vi "Get method name.vi"(8 "error in (no error)":errorcluster, 11 "VI in":refnum<vi>) -> (0 "error out":errorcluster, 1 "Body":T1, 3 "VI out":refnum<vi>)   [LabVIEW 2018]
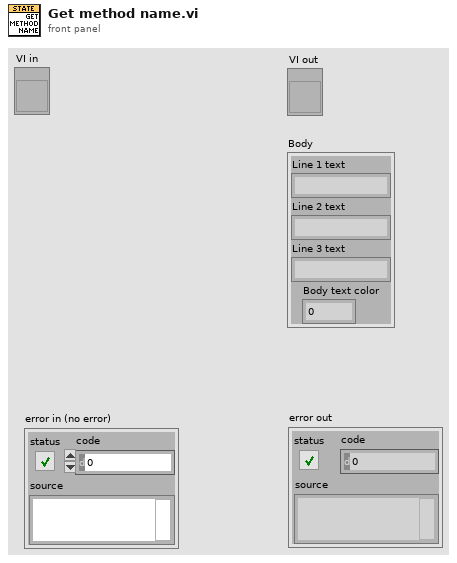
[diagram p1: front panel]
types:
  T1 = cluster{"Line 1 text":string, "Line 2 text":string, "Line 3 text":string, "Body text color":u32}
  T2 = cluster{"[0]":string, "[1]":string, "[2]":string}
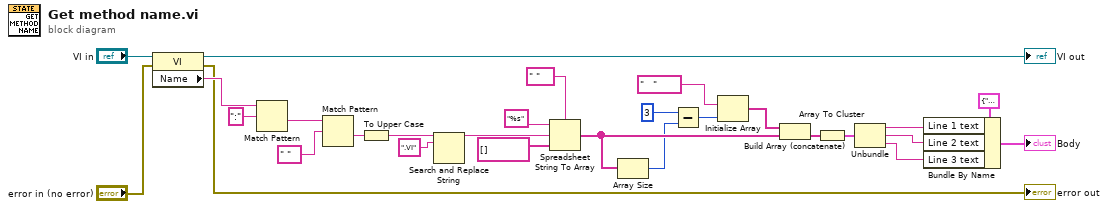
[diagram p0: block diagram]
diagram:
  n1 = property class="VI"(reference="VI in", error in="error in (no error)") -> (reference out=→"VI out":refnum<vi>, error out=→"error out":errorcluster, "Name"=w17:string)
  n2 = Match Pattern(string=w17, regular expression=":") -> (after substring=w19:string)  [unwired: 1 in, 3 out]
  n3 = Match Pattern(string=w19, regular expression=" ") -> (after substring=w20:string)  [unwired: 1 in, 3 out]
  n4 = To Upper Case(1:w20) -> (0:w22:string)
  n5 = Search and Replace String(input string=w22, search string=".VI") -> (result string=w27:string)  [unwired: 6 in, 3 out]
  n6 = Spreadsheet String To Array(delimiter (Tab)=" " ("search string"), format string="%s", spreadsheet string=w27, array type (2D Dbl)=string[] []) -> (array=w11:string[])
  n7 = Array Size(array=w11) -> (size(s)=w5:i32)
  n8 = Subtract(x=3, y=w5) -> (x-y=w4:i32)
  n9 = Initialize Array("   " ("search string"), w4) -> (w1:string[])
  n10 = Build Array (concatenate)(w1, w11) -> (w2:string[])
  n11 = Array To Cluster(array=w2) -> (cluster=w10:T2)
  n12 = Unbundle(w10) -> ("[0]"=w9:string, "[1]"=w8:string, "[2]"=w7:string)
  n13 = Bundle By Name(cluster=T1 {"Line 1 text"="", "Line 2 text"="", "Line 3 text"="", "Body text color"=0} ("Body"), "Line 1 text"=w9, "Line 2 text"=w8, "Line 3 text"=w7) -> (→"Body":T1)
